vi "更新程序.vi"() -> ()   [LabVIEW 2016, in "数据传输系统.lvlib"]
panel:
  out "waittime":u8
  out "端口号":i32
  out "IP地址":string
  out "步骤":string
  out "枚举":T1(ring)
  in  "目标路径（使用对话框）":path
  out "下载保存目录":path
  out "更新进度":u8(slide) scale=0.0..100.0
  # "1.先下载更新-------2.关闭主应用-------3.替换应用--------4.打开主应用-----------5.关闭本程序"
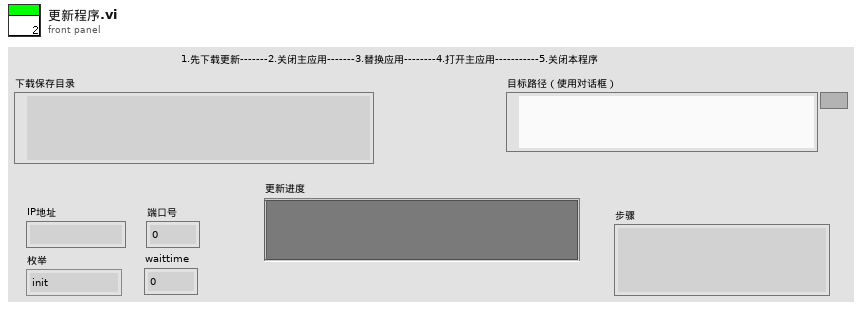
[diagram p1: front panel]
types:
  T1 = enum16{"init", "download", "close", "replace", "open", "over"}
  T2 = cluster{"网络灯":bool, "接收中":bool, "已接收百分比":u8, "接收成功次数":dbl, "当前步骤":enum16{"init", "receivehead", "receivecontent", "receivesuccess", "over"}, "error out":errorcluster}
  T3 = enum32{"Bad", "Idle", "Run top level", "Running"}
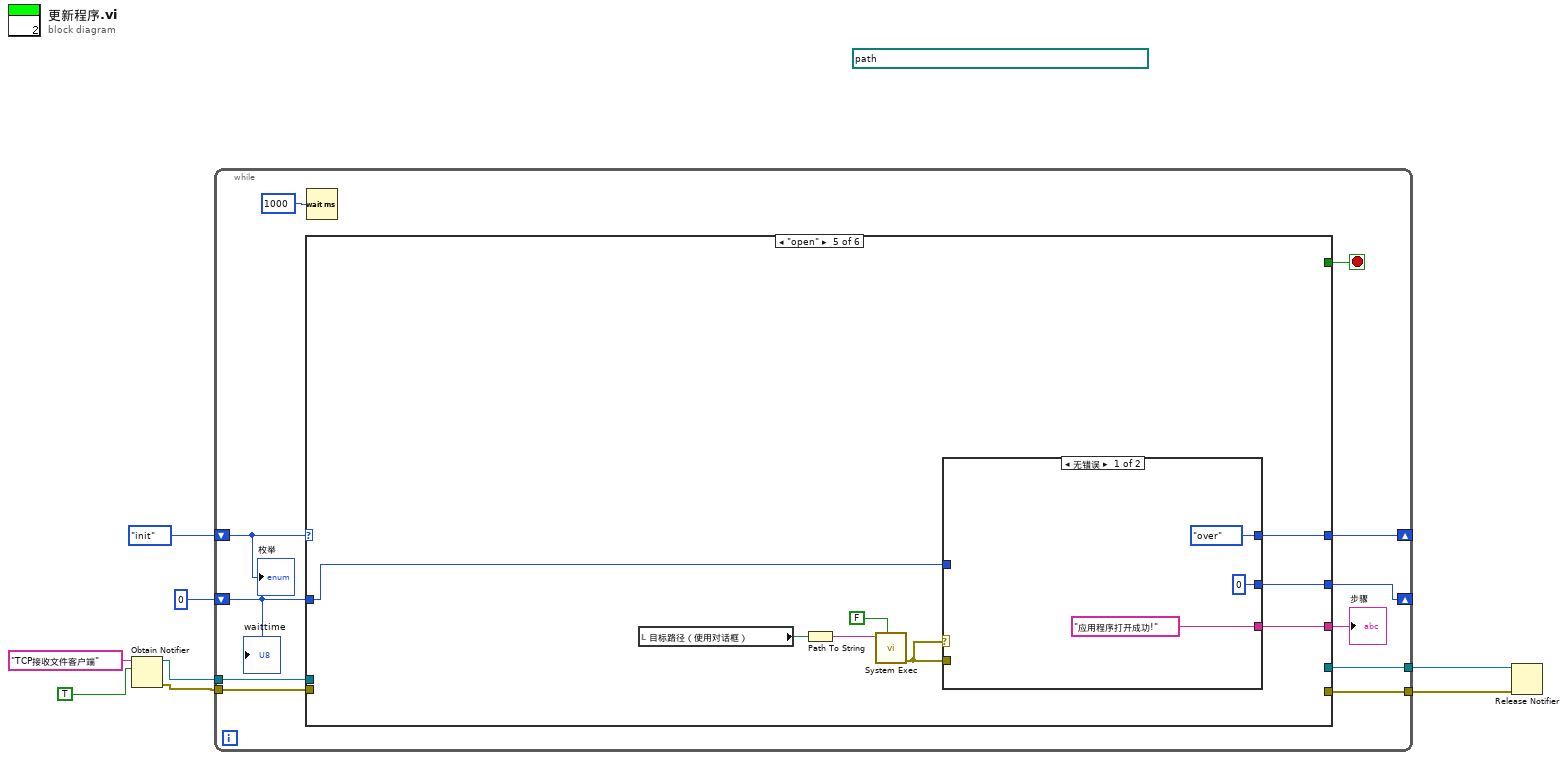
[diagram p0: block diagram]
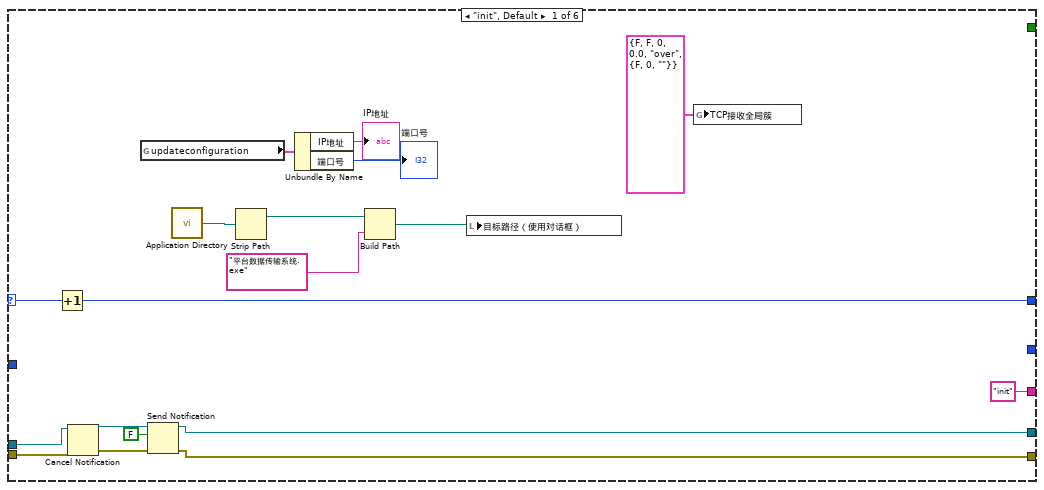
[diagram p2: hidden frame]
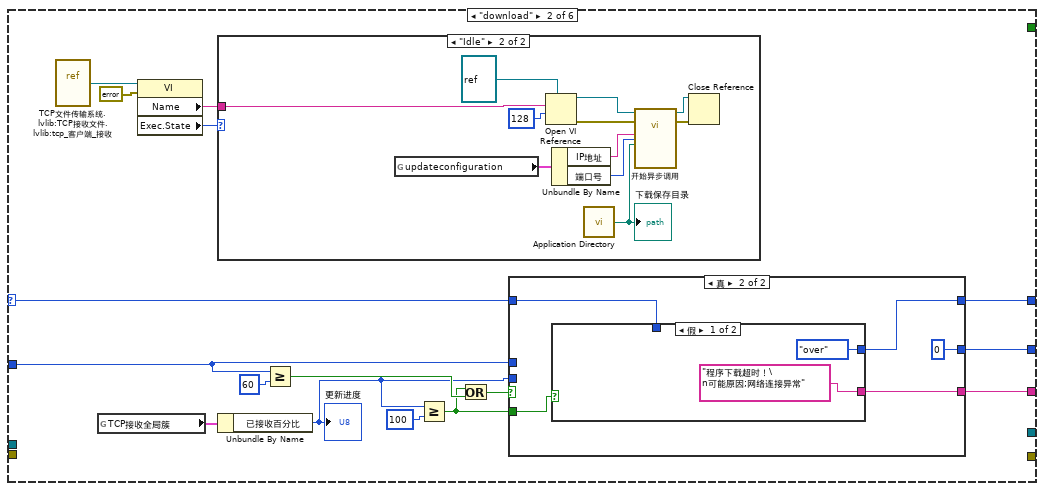
[diagram p3: hidden frame]
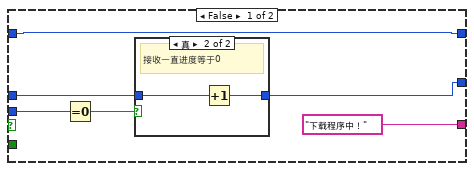
[diagram p5: hidden frame]
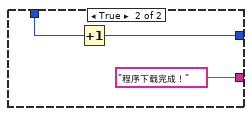
[diagram p7: hidden frame]
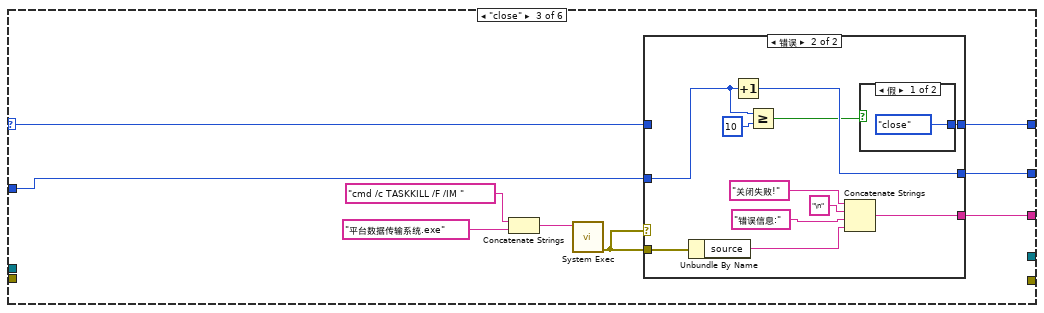
[diagram p8: hidden frame]
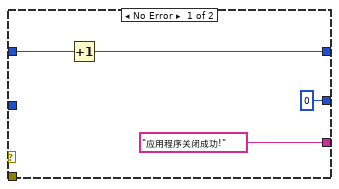
[diagram p9: hidden frame]
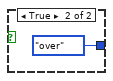
[diagram p10: hidden frame]
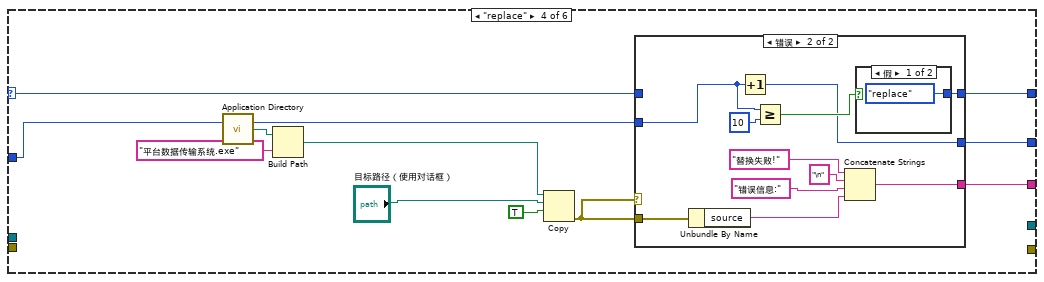
[diagram p11: hidden frame]
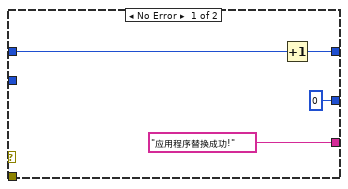
[diagram p12: hidden frame]
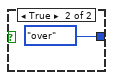
[diagram p13: hidden frame]
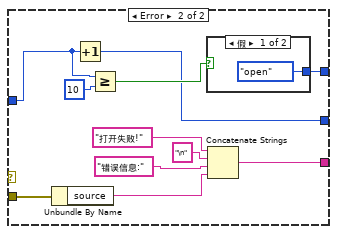
[diagram p14: hidden frame]
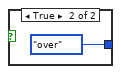
[diagram p15: hidden frame]
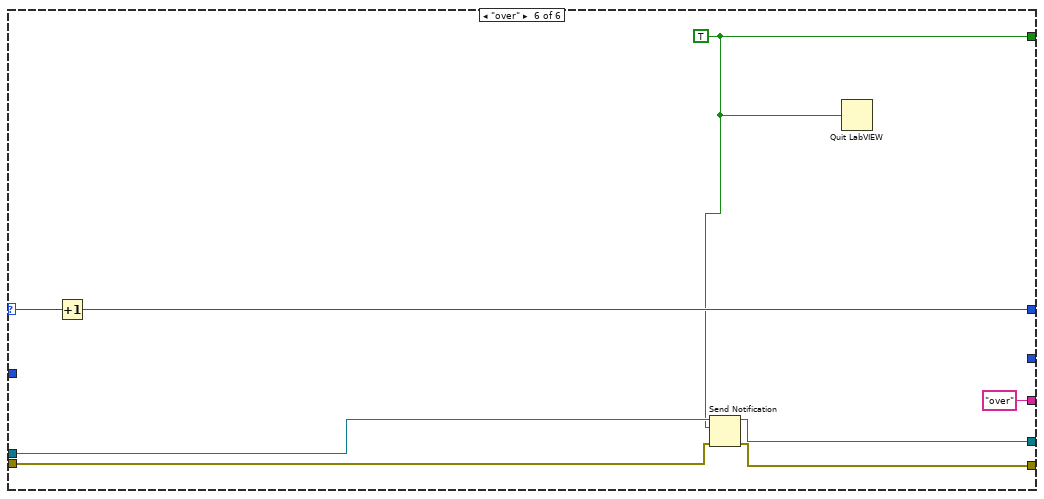
[diagram p16: hidden frame]
diagram:
  (unwired) path "C:/LabVIEW Project/builds/NEW平台数据传输系统"
  n1 = Obtain Notifier(name (unnamed)="TCP接收文件客户端" ("名称（未命名）"), notification data type=TRUE) -> (notifier out=w4:refnum<notifier>, error out=w3:errorcluster)  [unwired: 2 in, 1 out]
  n2 = while {
    shift-right: [w18] -> _
    shift-left: T1."init" -> [w19]
    shift-right: [w13] -> _
    shift-left: u8 0 ("y") -> [w14]
    tunnel: w4 -> [w12]
    tunnel: w3 -> [w11]
    tunnel: [w10] -> w2
    tunnel: [w9] -> w1
    stop <- w17 stop-if-true
    n3 = case shown="\"open\"" w19 {
      selector: w19 -> [w37 w46 w88 w118 _ w169]
      tunnel: [w36 w47 w87 w117 w141 w168] -> w18
      tunnel: [_ _ _ _ _ w162] -> w17
      tunnel: ["init" ("步骤") w43 w86 w116 w140 "over" ("步骤")] -> w15
      tunnel: w14 -> [_ w45 w85 w115 w139 _]
      tunnel: [_ w52 w84 w114 w138 _] -> w13
      tunnel: w12 -> [w27 _ _ _ _ w166]
      tunnel: w11 -> [w26 _ _ _ _ w165]
      tunnel: [w22 _ _ _ _ w164] -> w10
      tunnel: [w21 _ _ _ _ w163] -> w9
      frame "init", Default {
        n4 = Increment(x=w37) -> (x+1=w36:T1)
        n5 = Cancel Notification(0:w27, 3:w26) -> (8:w25:refnum<notifier>, 11:w23:errorcluster)  [unwired: 1 out]
        n6 = global read "断电保存全局.vi" "updateconfiguration"() -> (w34:cluster{"IP地址":string, "端口号":i32})
        n7 = Send Notification(notification=FALSE ("通知"), notifier=w25, error in (no error)=w23) -> (notifier out=w22:refnum<notifier>, error out=w21:errorcluster)
        n8 = call <vilib>:"Application Directory.vi"() -> ("Application Directory"=w31:path)
        n9 = Strip Path(path=w31) -> (stripped path=w30:path)  [unwired: 1 out]
        n10 = Unbundle By Name(w34) -> ("IP地址"=→"IP地址":string, "端口号"=→"端口号":i32)
        n11 = Build Path(base path=w30, name or relative path="平台数据传输系统.exe" ("字符串")) -> (appended path=w28:path)
        n12 = local write "目标路径（使用对话框）"(w28) -> ()
        n13 = global write "全局变量1.vi" "TCP接收全局簇"(T2 {"网络灯"=FALSE, "接收中"=FALSE, "已接收百分比"=0, "接收成功次数"=0.0, "当前步骤"=enum."over", "error out"={"status"=FALSE, "code"=0, "source"=""}} ("TCP接收全局簇")) -> ()
      }
      frame "download" {
        n14 = vi-ref "TCP文件传输系统.lvlib:TCP接收文件.lvlib:tcp_客户端_接收.vi"() -> (w38:refnum<vi>)
        n15 = global read "全局变量1.vi" "TCP接收全局簇"() -> (w44:T2)
        n16 = property class="VI"(reference=w38, error in=errorcluster {"status"=FALSE, "code"=0, "source"=""} ("错误输出")) -> ("Name"=w39:string, "Exec.State"=w41:T3)  [unwired: 2 out]
        n17 = case shown="\"Idle\"" w41 {
          tunnel: w39 -> [_ w61]
          frame "Bad", Default {
          }
          frame "Idle" {
            n18 = global read "断电保存全局.vi" "updateconfiguration"() -> (w54:cluster{"IP地址":string, "端口号":i32})
            n19 = Open VI Reference(type specifier VI Refnum (for type only)=refnum<vi> refnum, vi path=w61, options=128 ("选项")) -> (vi reference=w59:refnum<vi>, error out=w57:errorcluster)  [unwired: 3 in]
            n20 = Unbundle By Name(w54) -> ("IP地址"=w62:string, "端口号"=w63:i32)
            n21 = call <vilib>:"Application Directory.vi"() -> ("Application Directory"=w64:path)
            "下载保存目录" <- w64
            n22 = call-by-ref "开始异步调用"(reference=w59, error in=w57, "IP地址"=w62, "端口号"=w63, "储存路径"=w64) -> (reference out=w55:refnum<vi>, error out=w56:errorcluster)  [unwired: 17 in]
            n23 = Close Reference(reference=w55, error in (no error)=w56) -> ()  [unwired: 1 out]
          }
        }
        n24 = Unbundle By Name(w44) -> ("已接收百分比"=w48:u8)
        "更新进度" <- w48
        n25 = Greater Or Equal?(x=w45, y=u8 60) -> (x >= y?=w50:bool)
        n26 = Greater Or Equal?(x=w48, y=u8 100) -> (x >= y?=w42:bool)
        n27 = Or(x=w42, y=w50) -> (x .or. y?=w49:bool)
        n28 = case shown="真" w49 {
          tunnel: w45 -> [w70 _]
          tunnel: [w69 u8 0] -> w52
          tunnel: w48 -> [w67 _]
          tunnel: [w66 w74] -> w47
          tunnel: w46 -> [w66 w75]
          tunnel: ["下载程序中！" w76] -> w43
          tunnel: w42 -> [_ w77]
          frame False {
            n29 = Equal To 0?(x=w67) -> (x = 0?=w68:bool)
            n30 = case shown="真" w68 {
              tunnel: w70 -> [w71 w73]
              tunnel: [w71 w72] -> w69
              frame False {
              }
              frame True {
                # "接收一直进度等于0"
                n31 = Increment(x=w73) -> (x+1=w72:u8)
              }
            }
          }
          frame True {
            n32 = case shown="假" w77 {
              tunnel: ["程序下载超时！\n可能原因;网络连接异常" "程序下载完成！"] -> w76
              tunnel: w75 -> [_ w82]
              tunnel: [T1."over" w81] -> w74
              frame False {
              }
              frame True {
                n33 = Increment(x=w82) -> (x+1=w81:T1)
              }
            }
          }
        }
      }
      frame "close" {
        n34 = Concatenate Strings("cmd /c TASKKILL /F /IM " ("command line"), "平台数据传输系统.exe") -> (w89:string)
        n35 = call <vilib>:"System Exec.vi"("command line"=w89) -> ("error out"=w91:errorcluster)  [unwired: 7 in, 3 out]
        n36 = case shown="错误" w91 {
          tunnel: [w94 w101] -> w87
          tunnel: w91 -> [_ w107]
          tunnel: ["应用程序关闭成功!" ("步骤") w102] -> w86
          tunnel: w88 -> [w95 _]
          tunnel: w85 -> [_ w97]
          tunnel: [u8 0 w99] -> w84
          frame No Error {
            n37 = Increment(x=w95) -> (x+1=w94:T1)
          }
          frame Error {
            n38 = Unbundle By Name(w107) -> ("source"=w106:string)
            n39 = Increment(x=w97) -> (x+1=w99:u8)
            n40 = Greater Or Equal?(x=w97, y=u8 10) -> (x >= y?=w98:bool)
            n41 = Concatenate Strings("关闭失败!" ("消息"), "\n" ("字符串"), "错误信息:" ("字符串"), w106) -> (w102:string)
            n42 = case shown="假" w98 {
              tunnel: [T1."close" T1."over"] -> w101
              frame False {
              }
              frame True {
              }
            }
          }
        }
      }
      frame "replace" {
        n43 = call <vilib>:"Application Directory.vi"() -> ("Application Directory"=w112:path)
        n44 = Build Path(base path=w112, name or relative path="平台数据传输系统.exe" ("名称或相对路径")) -> (appended path=w110:path)
        n45 = Copy(9:TRUE ("覆盖(F)"), 10:"目标路径（使用对话框）", 11:w110) -> (0:w119:errorcluster)  [unwired: 2 in, 2 out]
        n46 = case shown="错误" w119 {
          tunnel: [w122 w129] -> w117
          tunnel: w119 -> [_ w135]
          tunnel: ["应用程序替换成功!" ("步骤") w130] -> w116
          tunnel: w118 -> [w123 _]
          tunnel: w115 -> [_ w127]
          tunnel: [u8 0 w125] -> w114
          frame No Error {
            n47 = Increment(x=w123) -> (x+1=w122:T1)
          }
          frame Error {
            n48 = Unbundle By Name(w135) -> ("source"=w134:string)
            n49 = Increment(x=w127) -> (x+1=w125:u8)
            n50 = Greater Or Equal?(x=w127, y=u8 10) -> (x >= y?=w126:bool)
            n51 = Concatenate Strings("替换失败!" ("消息"), "\n" ("字符串"), "错误信息:" ("字符串"), w134) -> (w130:string)
            n52 = case shown="假" w126 {
              tunnel: [T1."replace" T1."over"] -> w129
              frame False {
              }
              frame True {
              }
            }
          }
        }
      }
      frame "open" {
        n53 = local read "目标路径（使用对话框）"() -> (w142:path)
        n54 = Path To String(path=w142) -> (string=w145:string)
        n55 = call <vilib>:"System Exec.vi"("wait until completion? (T)"=FALSE, "command line"=w145) -> ("error out"=w143:errorcluster)  [unwired: 6 in, 3 out]
        n56 = case shown="无错误" w143 {
          tunnel: [T1."over" w153] -> w141
          tunnel: w143 -> [_ w159]
          tunnel: ["应用程序打开成功!" ("步骤") w154] -> w140
          tunnel: w139 -> [_ w151]
          tunnel: [u8 0 w149] -> w138
          frame No Error {
          }
          frame Error {
            n57 = Unbundle By Name(w159) -> ("source"=w158:string)
            n58 = Increment(x=w151) -> (x+1=w149:u8)
            n59 = Greater Or Equal?(x=w151, y=u8 10) -> (x >= y?=w150:bool)
            n60 = case shown="假" w150 {
              tunnel: [T1."open" T1."over"] -> w153
              frame False {
              }
              frame True {
              }
            }
            n61 = Concatenate Strings("打开失败!" ("消息"), "\n" ("字符串"), "错误信息:" ("字符串"), w158) -> (w154:string)
          }
        }
      }
      frame "over" {
        w162 = TRUE
        n62 = Increment(x=w169) -> (x+1=w168:T1)
        n63 = Send Notification(notification=w162, notifier=w166, error in (no error)=w165) -> (notifier out=w164:refnum<notifier>, error out=w163:errorcluster)
        n64 = Quit LabVIEW(quit? (T)=w162) -> ()
      }
    }
    "步骤" <- w15
    n65 = Wait (ms)(milliseconds to wait=u32 1000 ("等待时间（毫秒）")) -> ()  [unwired: 1 out]
    "枚举" <- w19
    "waittime" <- w14
  }
  n66 = Release Notifier(notifier=w2, error in (no error)=w1) -> ()  [unwired: 1 in, 3 out]
